vi "PyLoN_SRS4.vi"() -> ()   [LabVIEW 2014]
uses:
  <vilib>/Utility/file.llb/Write To Spreadsheet File (I64).vi
  <vilib>/Utility/file.llb/Write To Spreadsheet File (DBL).vi
panel:
  in  "CHEK ID":bool
  out "Max Value":dbl
  out "Min Value":dbl
  in  "Param ID":u32
  out "default value":dbl
  out "current value":dbl
  out "num of elements":dbl
  in  "?":bool
  in  "?":T1(tab)
  in  "Shutter State":u16(ring)=2 items=["Always Close", "Open Each Exposure", "Open Until Finish", "Open waiting for triger"]
  in  "Trigger Edge":u16(ring) items=["Positive", "Negative"]
  in  "Timing Mode":u16(ring) items=["Free Run", "Triger First", "Ext Sync", "Bulb Mode", "Variable Mode", "Flash Mode"]
  in  "ADC Speed":u16(ring)=2 items=["ADC Slowest", "ADC Fastest", "Default", "50 kHz", "100 kHz", "200 kHz", "500 kHz", "1 MHz"]
  in  "ADC Gain":u16(ring) items=["ADC Low", "ADC High"]
  in  "Temperature":dbl=-100.0 caption="SET Temperature" format="%.2f"
  in  "Skip Serial  Reg Clean":dbl=1.0 format="%.2f"
  in  "Vertical Timing":dbl=3.2
  out "Vertical Timing":dbl
  in  "Readout Port":i32=4 min=-1 step=1
  in  "?":T2={"X start"=0, "X end"=1023, "X Binning/Grouping"=1, "Y start"=0, "Y end"=1, "Y Binning/Grouping"=1}
  in  "Logic Out":u16(ring) items=["Not Scan", "Shutter", "Not Rady", "Logic 0", "Clearing", "Not Ft Image Shift", "Reserved", "Logic1", "Expos Prog", "Expos", "Image Shift", "Readout", "Acquiring", "Wait For Trig"]
  in  "Use Custom Chip":bool
  out "Readout Time":dbl caption="Readout time (ms)" format="%.2f"
  in  "Temp_bypass":bool
  in  "?":bool
  in  "Exposure Time (s)":dbl=0.004 min=0.0 step=0.001 format="%.3f"
  in  "?":bool
  in  "?":bool
  out "?":u16[](graph)
  in  "file path":path
  in  "File_name":string
  in  "# of spectrum per frame":i32
  in  "# of Frames":i32
  in  "FLIP SPECTRA":bool
  in  "?":bool
  in  "?":bool
  in  "?":bool
  out "?":dbl[](graph)
  in  "?":bool
  in  "Number of Images":u32=1 min=1 step=1
  out "?":dbl[](graph)
  in  "?":bool
  in  "# of Sets":i32
  out "Current Set":u32=24
  in  "#Ground per set":u32=3
  in  "Timepoints":dbl[](array[numeric])=[200.0, 100.0, 300.0, 400.0, 500.0]
  in  "File Path":path
  in  "File Name":string
  in  "Ground State\nSubstract?":bool
  in  "PyLonN Error In":errorcluster
  out "PyLoN Error Out":errorcluster
  out "PyLoN Ready":bool
  out "PyLoN \nTemperature":dbl
  # "REGION OF INTEREST"
  # "TRIGGER"
  # "ADC"
  # "SHUTTER"
  # "INPUT VARIABLES"
  # "TTL LOGIC"
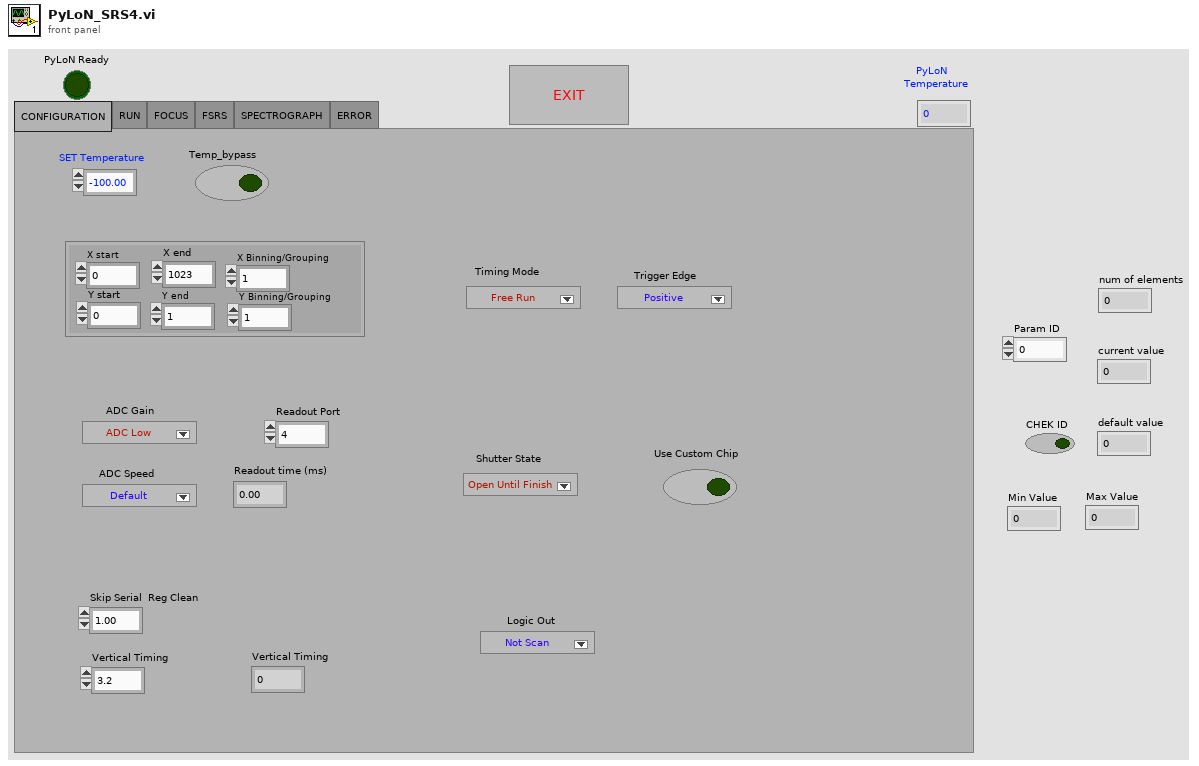
[diagram p1: front panel]
types:
  T1 = enum32{"CONFIGURATION", "RUN", "FOCUS", "FSRS", "SPECTROGRAPH", "ERROR"}
  T2 = cluster{"X start":u32, "X end":u32, "X Binning/Grouping":u32, "Y start":u32, "Y end":u32, "Y Binning/Grouping":u32}
  T3 = enum32{"Initializing", "RUN", "FSRS", "Monochromator", "Errors"}
  T4 = cluster{"Param ID":u32, "Avail Flag":u8, "Current Value":dbl, "Default Value":dbl, "Min Value":dbl, "Max Value":dbl, "Increment":dbl, "Data Type":u32, "Access Type":u32, "Bit Used Flag":u32, "Number of Enums":u32, "Description":string}
  T5 = cluster{"acquire focus mode":u32, "Exposure Time (s)":dbl, i32, "Software accumulation":u32}
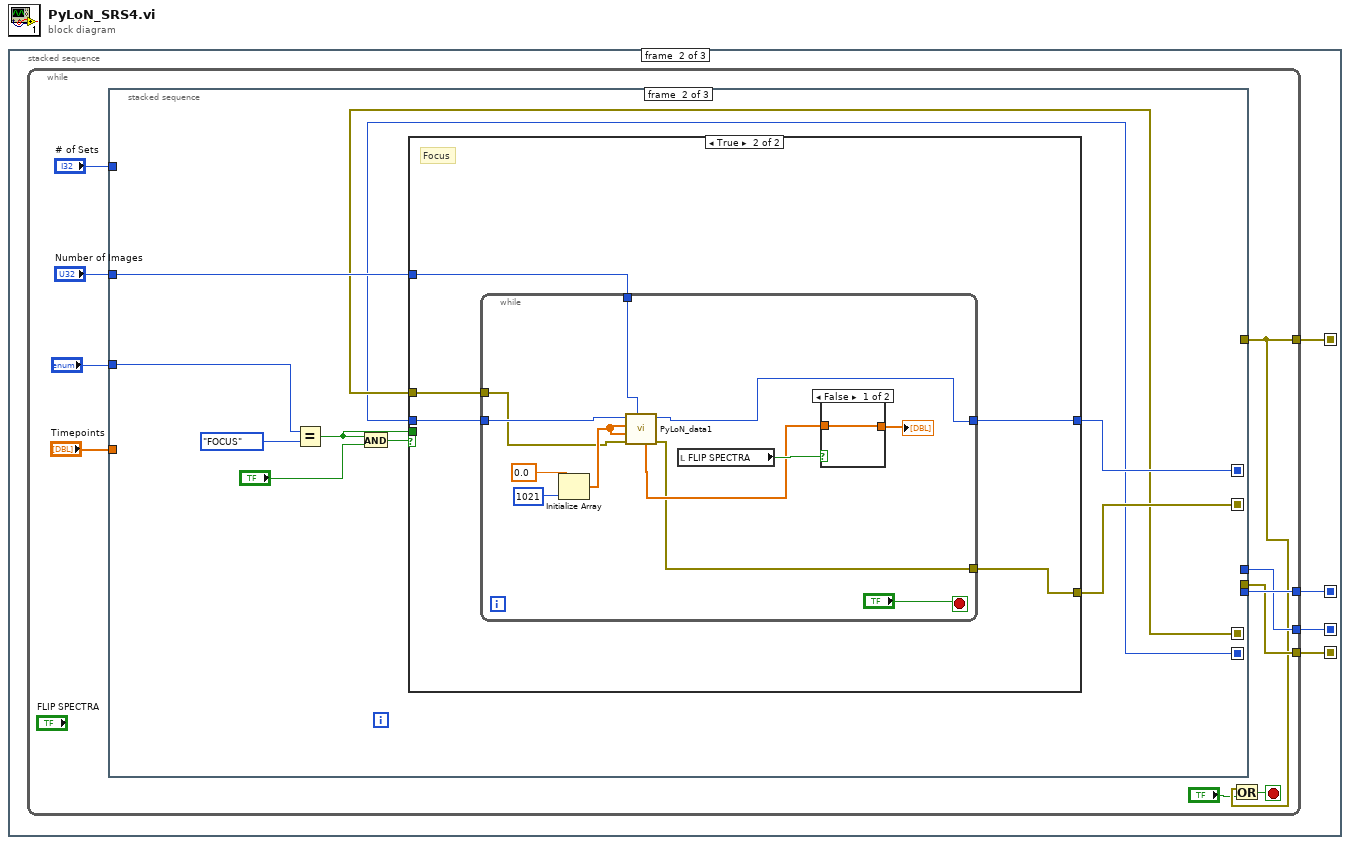
[diagram p0: block diagram]
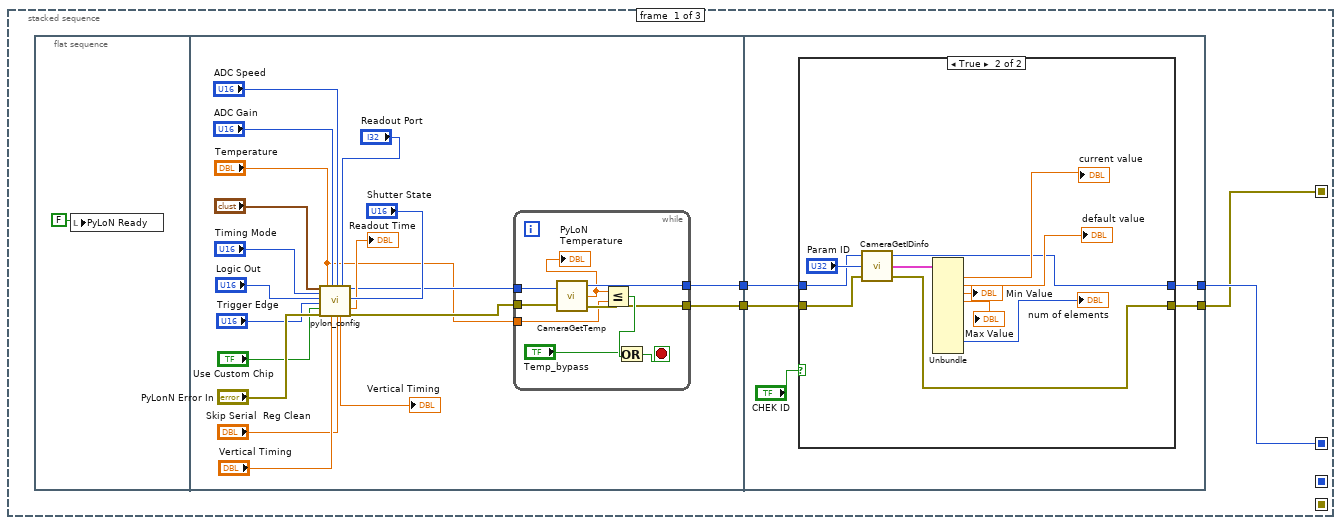
[diagram p2: hidden frame]
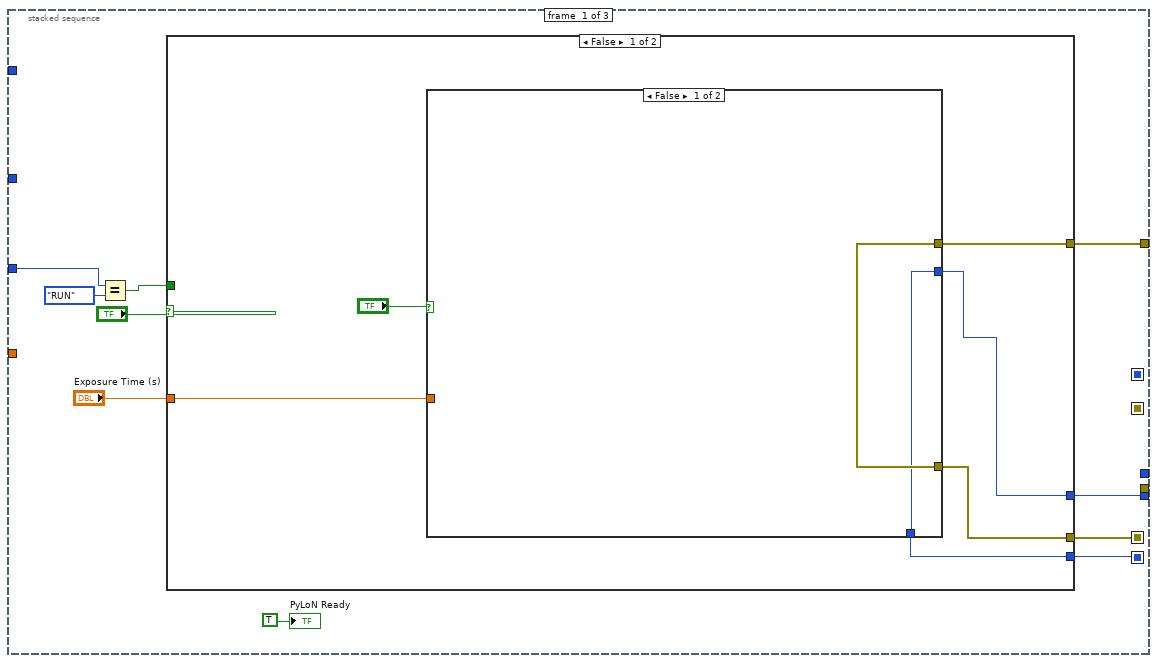
[diagram p4: hidden frame]
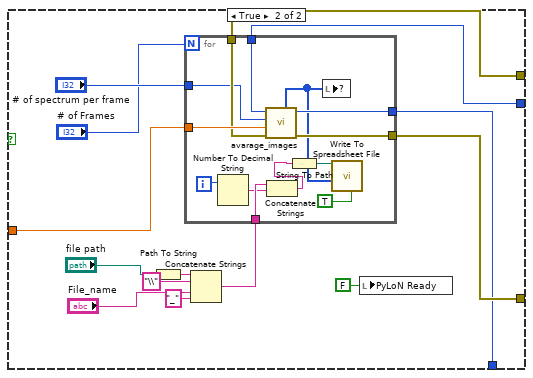
[diagram p5: hidden frame]
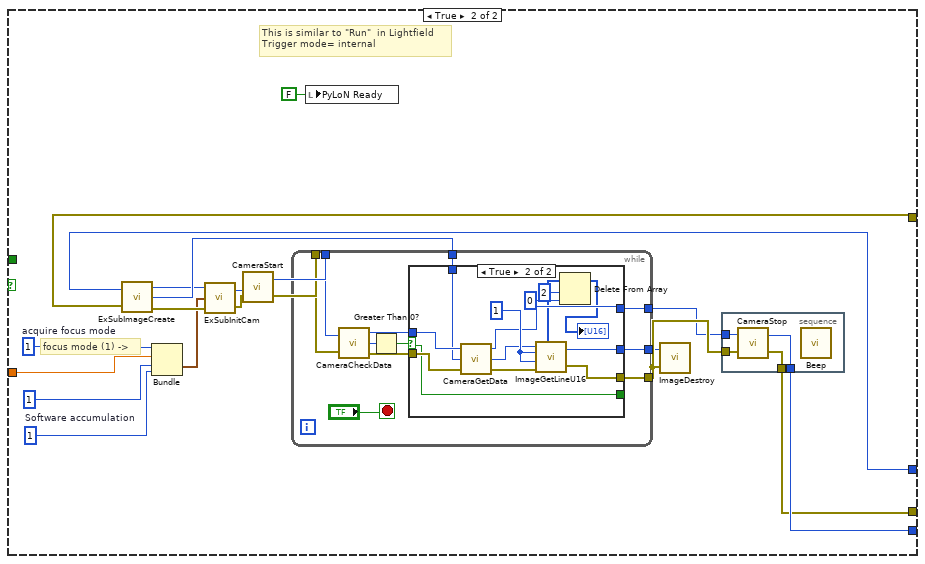
[diagram p6: hidden frame]
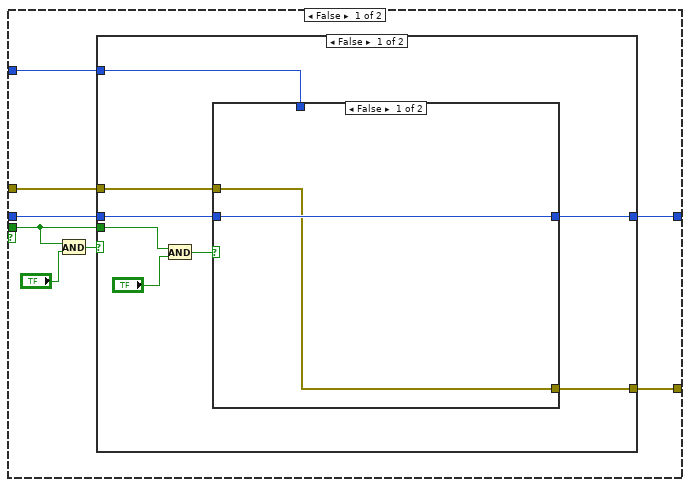
[diagram p8: hidden frame]
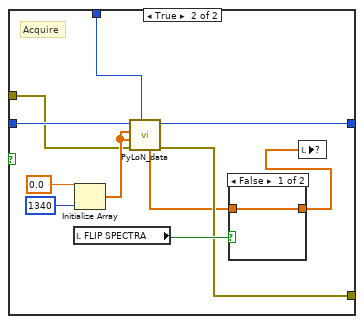
[diagram p9: hidden frame]
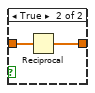
[diagram p10: hidden frame]
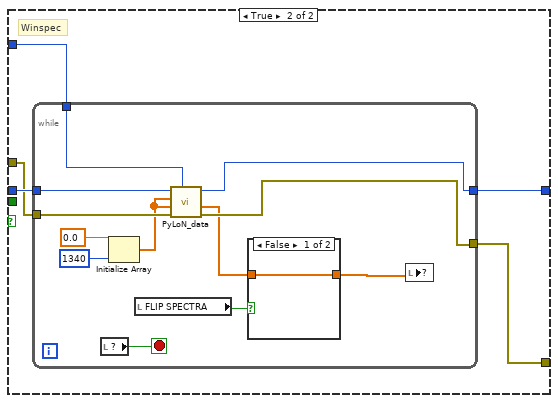
[diagram p11: hidden frame]
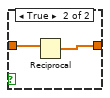
[diagram p12: hidden frame]
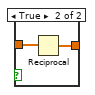
[diagram p13: hidden frame]
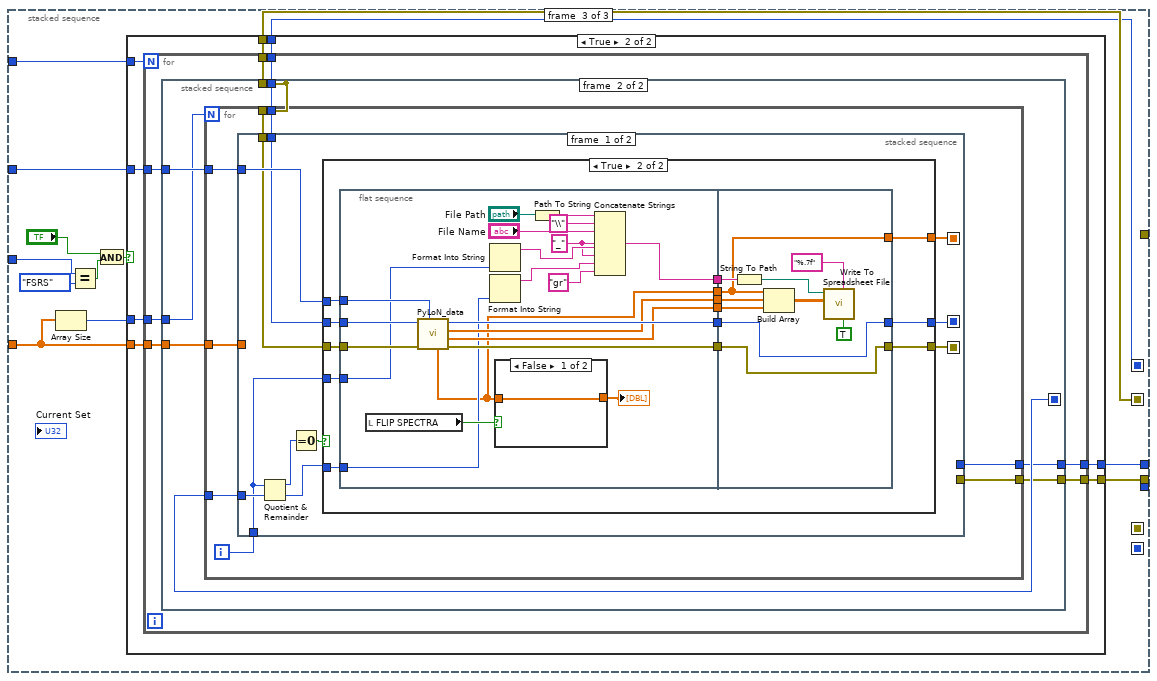
[diagram p14: hidden frame]
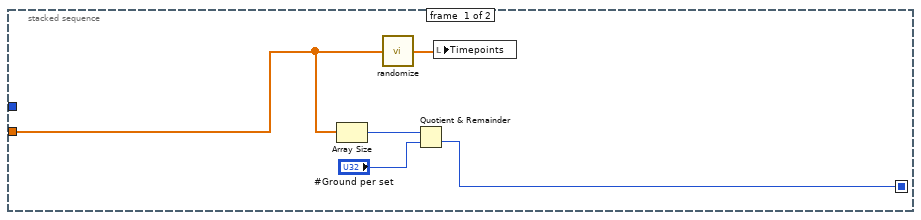
[diagram p16: hidden frame]
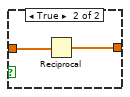
[diagram p18: hidden frame]
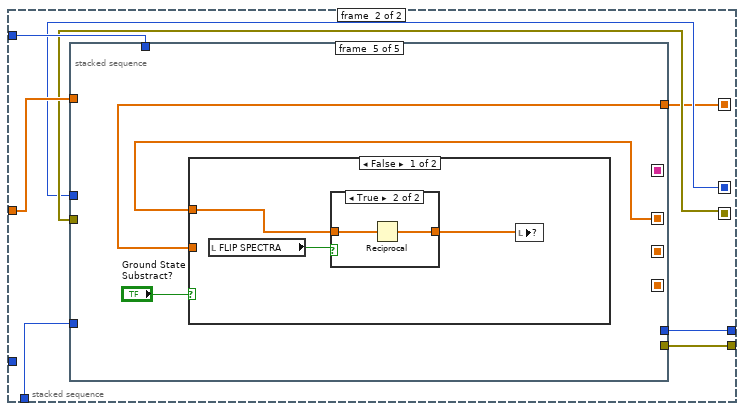
[diagram p19: hidden frame]
diagram:
  n1 = stacked-sequence {
    seq-local: [w3 _ _] -> [_ w52 _]
    seq-local: [w4 _ _] -> [_ w55 _]
    seq-local: [_ w54 _] -> [_ _ w416]
    seq-local: [_ w53 _] -> [_ _ w415]
    frame #0 {
      n2 = flat-sequence {
        tunnel: [w9] -> w2
        tunnel: [w7] -> w1
        tunnel: [w34] -> w3
        tunnel: [w37] -> w4
        tunnel: w2 -> [w38]
        tunnel: w1 -> [w36]
        frame #0 {
          n3 = local write "PyLoN Ready"(FALSE ("PyLoN Ready")) -> ()
        }
        frame #1 {
          n4 = call "pylon_config.vi"(0:"?", "Timing Mode"="Timing Mode", "Logic Out"="Logic Out", "Trigger Edge"="Trigger Edge", "Use Custom Chip"="Use Custom Chip", "PyLonN Error In"="PyLonN Error In", "Temperature"="Temperature", "ADC Gain"="ADC Gain", "Vertical Timing"="Vertical Timing", "ADC Speed"="ADC Speed", "Skip Serial  Reg Clean"="Skip Serial  Reg Clean", "Readout Port"="Readout Port", "Shutter State"="Shutter State") -> ("Vertical Timing"=→"Vertical Timing":dbl, "CameraHandle"=w10:u32, "Readout Time"=→"Readout Time":dbl, "error out"=w8:errorcluster)  [unwired: 3 in]
          n5 = while {
            tunnel: [w33] -> w9
            tunnel: w10 -> [w30]
            tunnel: w8 -> [w29]
            tunnel: [w28] -> w7
            tunnel: "Temperature" -> [w26]
            stop <- w32 stop-if-true
            n6 = call <userlib>:"CameraGetTemp.vi"("Camera Handle"=w30, "error in (no error)"=w29) -> ("Camera Handle"=w33:u32, "Temperature"=w27:dbl, "error out"=w28:errorcluster)
            "PyLoN \nTemperature" <- w27
            n7 = Less Or Equal?(x=w27, y=w26) -> (x <= y?=w31:bool)
            n8 = Or(x="Temp_bypass", y=w31) -> (x .or. y?=w32:bool)
          }
        }
        frame #2 {
          n9 = case shown="True" "CHEK ID" {
            tunnel: w38 -> [w40 w46]
            tunnel: [w40 w45] -> w37
            tunnel: w36 -> [w39 w44]
            tunnel: [w39 w43] -> w34
            frame False {
            }
            frame True {
              n10 = call <userlib>:"CameraGetIDinfo.vi"("error in"=w44, "Param ID"="Param ID", "Camera handle"=w46) -> ("error out"=w43:errorcluster, "Param ID Information"=w51:T4, "Camera handle"=w45:u32)
              n11 = Unbundle(w51) -> ("Current Value"=→"current value":dbl, "Default Value"=→"default value":dbl, "Min Value"=→"Min Value":dbl, "Max Value"=→"Max Value":dbl, "Number of Enums"=→"num of elements":u32)  [unwired: 7 out]
            }
          }
        }
      }
    }
    frame #1 {
      n12 = while {
        tunnel: w55 -> [w65]
        tunnel: w52 -> [w57]
        tunnel: [w61] -> w54
        tunnel: [w60] -> w53
        stop <- w58 stop-if-true
        n13 = stacked-sequence {
          seq-local: [_ w168 _] -> [_ _ w252]
          seq-local: [_ w167 _] -> [_ _ w254]
          seq-local: [w70 _ _] -> [_ w165 _]
          seq-local: [w71 _ _] -> [_ w166 _]
          tunnel: w65 -> [w68 _ _]
          tunnel: w57 -> [w75 _ _]
          tunnel: "?" -> [w72 w173 w258]
          tunnel: "Number of Images" -> [_ w171 w255]
          tunnel: "Timepoints" -> [_ _ w247]
          tunnel: [_ _ w251] -> w61
          tunnel: [_ _ w250] -> w60
          tunnel: "# of Sets" -> [_ _ w248]
          frame #0 {
            n14 = Equal?(x=w72, y=T3."RUN") -> (x = y?=w69:bool)
            n15 = case shown="False" "?" {
              tunnel: w75 -> [w81 w113]
              tunnel: [w78 w116] -> w70
              tunnel: [w80 w115] -> w71
              tunnel: w69 -> [_ _]
              tunnel: w68 -> [w79 w114]
              tunnel: "Exposure Time (s)" -> [w77 w111]
              frame False {
                n16 = case shown="False" "?" {
                  tunnel: w81 -> [w83 w95]
                  tunnel: [w83 w94] -> w80
                  tunnel: w79 -> [w82 w96]
                  tunnel: [w82 w93] -> w78
                  tunnel: w77 -> [_ w97]
                  frame False {
                  }
                  frame True {
                    n17 = Path To String(path="file path") -> (string=w89:string)
                    n18 = Concatenate Strings(w89, "\\" ("string"), "File_name", "_" ("string")) -> (w84:string)
                    n19 = for {
                      N: "# of Frames" -> [_]
                      tunnel: w97 -> [w110]
                      tunnel: w96 -> [w109]
                      tunnel: w95 -> [w108]
                      tunnel: [w107] -> w94
                      tunnel: [w106] -> w93
                      tunnel: "# of spectrum per frame" -> [w105]
                      tunnel: w84 -> [w101]
                      i -> [w98]
                      n20 = Number To Decimal String(number=w98) -> (decimal integer string=w100:string)  [unwired: 1 in]
                      n21 = call "avarage_images.vi"("error in (no error)"=w108, "Exposure Time (s)"=w110, "Number of Images"=w105, "Camera Handle"=w109) -> ("error out"=w107:errorcluster, "Camera Handle"=w106:u32, "Waveform Graph"=w104:i32[])  [unwired: 3 in, 2 out]
                      n22 = Concatenate Strings(w101, w100) -> (w99:string)
                      n23 = String To Path(string=w99) -> (path=w102:path)
                      n24 = local write item#9(w104) -> ()
                      n25 = call-poly <vilib>:"Write To Spreadsheet File.vi"("transpose? (no:F)"=TRUE, "1D data"=w104, "file path (dialog if empty)"=w102) -> ()  [unwired: 5 in, 1 out]
                    }
                    n26 = local write "PyLoN Ready"(FALSE ("PyLoN Ready")) -> ()
                  }
                }
              }
              frame True {
                w118 = u32 1  # acquire focus mode
                w119 = u32 1  # Software accumulation
                # "focus mode (1) ->"
                # "This is similar to \"Run\"  in Lightfield\nTrigger mode= internal"
                n27 = call "ExSubImageCreate.vi"("Camera Handle"=w114, "error in (no error)"=w113) -> ("Camera Handle"=w120:u32, "Data Handle"=w126:u32, "error out"=w121:errorcluster)
                n28 = Bundle("acquire focus mode"=w118, "Exposure Time (s)"=w111, 1, "Software accumulation"=w119) -> (w117:T5)  [unwired: 1 in]
                n29 = call "ExSubInitCam.vi"("error in (no error)"=w121, "Camera Information"=w117, "Camera Handle"=w120) -> ("error out"=w122:errorcluster, "Camera Handle"=w123:u32)
                n30 = call <userlib>:"CameraStart.vi"("error in"=w122, "Camera Handle"=w123) -> ("error out"=w124:errorcluster, "Camera Handle"=w125:u32)
                n31 = while {
                  tunnel: [w141] -> w127
                  tunnel: [w140] -> w129
                  tunnel: [w139] -> w128
                  tunnel: w124 -> [w138]
                  tunnel: w125 -> [w137]
                  tunnel: w126 -> [w136]
                  stop <- "?" stop-if-true
                  n32 = call <userlib>:"CameraCheckData.vi"("Camera Handle"=w137, "error in"=w138) -> ("Camera Handle"=w143:u32, "Number Of Frames Available"=w145:i32, "error out"=w142:errorcluster)
                  n33 = Greater Than 0?(x=w145) -> (x > 0?=w144:bool)
                  n34 = case shown="True" w144 {
                    selector: w144 -> [w148 w161]
                    tunnel: w143 -> [w146 w163]
                    tunnel: w142 -> [w149 w162]
                    tunnel: [w148 w161] -> _
                    tunnel: [w149 w160] -> w140
                    tunnel: w136 -> [w147 w154]
                    tunnel: [w147 w158] -> w141
                    tunnel: [w146 w157] -> w139
                    frame False {
                    }
                    frame True {
                      w159 = 1
                      n35 = call <userlib>:"CameraGetData.vi"("error in"=w162, "Data Handle"=w154, "Camera Handle"=w163) -> ("error out"=w156:errorcluster, "Data Handle"=w155:u32, "Camera Handle"=w157:u32)
                      n36 = call <userlib>:"ImageGetLineU16.vi"("Data Handle"=w155, "Y Position"=w159, "Z Position"=w159, "error in"=w156) -> ("Array u16"=w153:u16[], "Data Handle"=w158:u32, "error out"=w160:errorcluster)
                      n37 = Delete From Array(array=w153, length=2, index=0) -> (array with subset deleted=→"?":u16[])  [unwired: 1 out]
                    }
                  }
                }
                n38 = local write "PyLoN Ready"(FALSE ("PyLoN Ready")) -> ()
                n39 = call <userlib>:"ImageDestroy.vi"("error in"=w129, "Data handle"=w127) -> ()  [unwired: 1 out]
                n40 = stacked-sequence {
                  tunnel: w129 -> [w134]
                  tunnel: w128 -> [w133]
                  tunnel: [w132] -> w115
                  tunnel: [w131] -> w116
                  frame #0 {
                    n41 = call <userlib>:"CameraStop.vi"("error in"=w134, "Camera Handle"=w133) -> ("error out"=w132:errorcluster, "Camera Handle"=w131:u32)
                    n42 = call <vilib>:"Beep.vi"() -> ()  [unwired: 12 in]
                  }
                }
              }
            }
            "PyLoN Ready" <- TRUE
          }
          frame #1 {
            n43 = Equal?(x=w173, y=T1."FOCUS") -> (x = y?=w169:bool)
            n44 = And(x=w169, y="?") -> (x .and. y?=w172:bool)
            n45 = case shown="True" w172 {
              tunnel: w165 -> [w181 w230]
              tunnel: [w177 w229] -> w168
              tunnel: w166 -> [w179 w228]
              tunnel: w171 -> [w180 w227]
              tunnel: [w178 w226] -> w167
              tunnel: w169 -> [w174 _]
              frame False {
                n46 = And(x=w174, y="?") -> (x .and. y?=w176:bool)
                n47 = case shown="False" w176 {
                  tunnel: w181 -> [w184 w210]
                  tunnel: w180 -> [w185 w209]
                  tunnel: w179 -> [w186 w208]
                  tunnel: [w182 w207] -> w178
                  tunnel: [w183 w206] -> w177
                  tunnel: w174 -> [w187 _]
                  frame False {
                    n48 = And(x=w187, y="?") -> (x .and. y?=w189:bool)
                    n49 = case shown="False" w189 {
                      tunnel: w186 -> [w190 w195]
                      tunnel: w185 -> [_ w198]
                      tunnel: w184 -> [w191 w197]
                      tunnel: [w191 w193] -> w183
                      tunnel: [w190 w194] -> w182
                      frame False {
                      }
                      frame True {
                        # "Acquire"
                        n50 = local read "FLIP SPECTRA"() -> (w200:bool)
                        n51 = Initialize Array(0.0, u32 1340) -> (w196:dbl[])
                        n52 = call "PyLoN_data.vi"("Number of Images"=w198, "error in (no error)"=w195, "PumpOffBkgd"=w196, "PumpOnBkgd"=w196, "Camera Handle"=w197) -> ("error out"=w194:errorcluster, "Camera Handle 2"=w193:u32, "Raman_Gain"=w192:dbl[])  [unwired: 2 in, 2 out]
                        n53 = case shown="False" w200 {
                          tunnel: w192 -> [w203 w205]
                          tunnel: [w203 w204] -> w199
                          frame False {
                          }
                          frame True {
                            n54 = Reciprocal(x=w205) -> (1/x=w204:dbl[])
                          }
                        }
                        n55 = local write item#21(w199) -> ()
                      }
                    }
                  }
                  frame True {
                    # "Winspec"
                    n56 = while {
                      tunnel: w210 -> [w216]
                      tunnel: w209 -> [w217]
                      tunnel: [w211] -> w206
                      tunnel: w208 -> [w215]
                      tunnel: [w214] -> w207
                      stop <- w220 stop-if-true
                      n57 = local read item#27() -> (w220:bool)
                      n58 = Initialize Array(0.0, u32 1340) -> (w212:dbl[])
                      n59 = local read "FLIP SPECTRA"() -> (w219:bool)
                      n60 = call "PyLoN_data.vi"("Number of Images"=w217, "error in (no error)"=w215, "PumpOffBkgd"=w212, "PumpOnBkgd"=w212, "Camera Handle"=w216) -> ("error out"=w214:errorcluster, "Pump_Off"=w213:dbl[], "Camera Handle 2"=w211:u32)  [unwired: 2 in, 2 out]
                      n61 = case shown="False" w219 {
                        tunnel: w213 -> [w223 w224]
                        tunnel: [w223 w225] -> w218
                        frame False {
                        }
                        frame True {
                          n62 = Reciprocal(x=w224) -> (1/x=w225:dbl[])
                        }
                      }
                      n63 = local write item#21(w218) -> ()
                    }
                  }
                }
              }
              frame True {
                # "Focus"
                n64 = while {
                  tunnel: w228 -> [w234]
                  tunnel: w227 -> [w237]
                  tunnel: [w232] -> w226
                  tunnel: w230 -> [w236]
                  tunnel: [w231] -> w229
                  stop <- "?" stop-if-true
                  n65 = Initialize Array(0.0, u32 1021) -> (w235:dbl[])
                  n66 = call "PyLoN_data1.vi"("Number of Images"=w237, "error in (no error)"=w234, "PumpOffBkgd"=w235, "PumpOnBkgd"=w235, "Camera Handle"=w236) -> ("error out"=w232:errorcluster, "Camera Handle 2"=w231:u32, "Raman_Gain"=w233:dbl[])  [unwired: 2 in, 2 out]
                  n67 = local read "FLIP SPECTRA"() -> (w239:bool)
                  n68 = case shown="False" w239 {
                    tunnel: w233 -> [w243 w245]
                    tunnel: [w243 w244] -> w238
                    frame False {
                    }
                    frame True {
                      n69 = Reciprocal(x=w245) -> (1/x=w244:dbl[])
                    }
                  }
                  "?" <- w238
                }
              }
            }
          }
          frame #2 {
            n70 = Array Size(array=w247) -> (size(s)=w246:i32)
            n71 = Equal?(x=w258, y=T1."FSRS") -> (x = y?=w256:bool)
            n72 = And(x="?", y=w256) -> (x .and. y?=w257:bool)
            n73 = case shown="True" w257 {
              tunnel: w255 -> [_ w268]
              tunnel: w252 -> [w259 w267]
              tunnel: w254 -> [w260 w263]
              tunnel: w247 -> [_ w266]
              tunnel: [w259 w265] -> w251
              tunnel: [w260 w264] -> w250
              tunnel: w248 -> [_ w262]
              tunnel: w246 -> [_ w261]
              frame False {
              }
              frame True {
                n74 = for {
                  N: w262 -> [_]
                  tunnel: w268 -> [w275]
                  tunnel: w267 -> [w274]
                  tunnel: w266 -> [w273]
                  tunnel: [w272] -> w265
                  tunnel: [w271] -> w264
                  tunnel: w263 -> [w270]
                  tunnel: w261 -> [w269]
                  n75 = stacked-sequence {
                    seq-local: [w278 _] -> [_ w288]
                    tunnel: w275 -> [_ w287]
                    tunnel: w274 -> [_ w286]
                    tunnel: [_ w282] -> _
                    tunnel: w273 -> [w276 w285]
                    tunnel: [_ w284] -> w271
                    tunnel: [_ w283] -> w272
                    tunnel: w270 -> [_ w282]
                    tunnel: w269 -> [_ w281]
                    frame #0 {
                      n76 = Array Size(array=w276) -> (size(s)=w280:i32)
                      n77 = call "randomize.vi"("Input array"=w276) -> ("Output array"=w277:dbl[])
                      n78 = Quotient & Remainder(x=w280, y="#Ground per set") -> (floor(x/y)=w278:u32)  [unwired: 1 out]
                      n79 = local write "Timepoints"(w277) -> ()
                    }
                    frame #1 {
                      n80 = for {
                        N: w281 -> [_]
                        tunnel: w288 -> [w295]
                        tunnel: w287 -> [w294]
                        tunnel: w286 -> [w293]
                        tunnel: w285 -> [w292]
                        tunnel: [w291] -> w284
                        tunnel: [w290] -> w283
                        tunnel: w282 -> [w289]
                        i -> [w296]
                        n81 = stacked-sequence {
                          seq-local: [w298 _] -> [_ w361]
                          seq-local: [w299 _] -> [_ w362]
                          seq-local: [w297 _] -> [_ w360]
                          tunnel: w296 -> [w300 w363]
                          tunnel: w295 -> [w305 _]
                          tunnel: w294 -> [w303 w365]
                          tunnel: w293 -> [w302 _]
                          tunnel: w289 -> [w301 _]
                          tunnel: w292 -> [_ w364]
                          tunnel: [_ w359] -> w291
                          tunnel: [_ w358] -> w290
                          frame #0 {
                            n82 = Quotient & Remainder(x=w300, y=w305) -> (x-y*floor(x/y)=w306:u32, floor(x/y)=w304:u32)
                            n83 = Equal To 0?(x=w306) -> (x = 0?=w307:bool)
                            n84 = case shown="True" w307 {
                              tunnel: w304 -> [_ w319]
                              tunnel: w303 -> [_ w323]
                              tunnel: w302 -> [w309 w322]
                              tunnel: w301 -> [w308 w321]
                              tunnel: [w309 w312] -> w298
                              tunnel: [w308 w311] -> w299
                              tunnel: w300 -> [_ w320]
                              tunnel: [_ w310] -> w297
                              frame False {
                              }
                              frame True {
                                n85 = flat-sequence {
                                tunnel: w323 -> [w344]
                                tunnel: w322 -> [w343]
                                tunnel: w321 -> [w342]
                                tunnel: w320 -> [w330]
                                tunnel: w319 -> [w328]
                                tunnel: [w341] -> w318
                                tunnel: [w340] -> w317
                                tunnel: [w337] -> w316
                                tunnel: [w336] -> w315
                                tunnel: [w325] -> w314
                                tunnel: [w324] -> w313
                                tunnel: w318 -> [w350]
                                tunnel: w317 -> [w349]
                                tunnel: w316 -> [w353]
                                tunnel: w315 -> [w352]
                                tunnel: w314 -> [w354]
                                tunnel: w313 -> [w348]
                                tunnel: [w350] -> w312
                                tunnel: [w349] -> w311
                                tunnel: [w348] -> w310
                                frame #0 {
                                w329 = "_" ("string")
                                n86 = local read "FLIP SPECTRA"() -> (w339:bool)
                                n87 = call "PyLoN_data.vi"("Number of Images"=w344, "error in (no error)"=w342, "Camera Handle"=w343) -> ("error out"=w340:errorcluster, "Pump_Off"=w336:dbl[], "Pump_On"=w337:dbl[], "Camera Handle 2"=w341:u32, "Raman_Gain"=w324:dbl[])  [unwired: 4 in]
                                n88 = Format Into String(w330) -> (resulting string=w331:string)  [unwired: 3 in, 1 out]
                                n89 = Format Into String(w328) -> (resulting string=w327:string)  [unwired: 3 in, 1 out]
                                n90 = case shown="False" w339 {
                                tunnel: w324 -> [w345 w347]
                                tunnel: [w345 w346] -> w338
                                frame False {
                                }
                                frame True {
                                n91 = Reciprocal(x=w347) -> (1/x=w346:dbl[])
                                }
                                }
                                "?" <- w338
                                n92 = Path To String(path="File Path") -> (string=w335:string)
                                n93 = Concatenate Strings(w335, "\\" ("string"), "File Name", w329, w331, w329, w327, "gr" ("string")) -> (w325:string)
                                }
                                frame #1 {
                                n94 = String To Path(string=w354) -> (path=w355:path)
                                n95 = Build Array(w348, w353, w352) -> (w351:dbl[][])
                                n96 = call-poly <vilib>:"Write To Spreadsheet File.vi"("transpose? (no:F)"=TRUE, "format (%.3f)"="%.7f", "2D data"=w351, "file path (dialog if empty)"=w355) -> ()  [unwired: 4 in, 1 out]
                                }
                                }
                              }
                            }
                          }
                          frame #1 {
                            n97 = stacked-sequence {
                              seq-local: [_ w368 _ _ _] -> [_ _ _ w389 _]
                              seq-local: [_ w371 _ _ _] -> [_ _ _ w388 w395]
                              seq-local: [_ w370 _ _ _] -> [_ _ _ w387 _]
                              seq-local: [_ w369 _ _ _] -> [_ _ _ w386 _]
                              tunnel: w362 -> [_ w381 _ _ _]
                              tunnel: w361 -> [_ w380 _ _ _]
                              tunnel: w365 -> [_ w379 _ _ _]
                              tunnel: w364 -> [_ w376 _ _ _]
                              tunnel: w363 -> [_ w372 _ _ _]
                              tunnel: w360 -> [_ _ _ _ w396]
                              tunnel: [_ w367 _ _ _] -> w359
                              tunnel: [_ w366 _ _ _] -> w358
                              frame #0 {
                              }
                              frame #1 {
                                n98 = Index Array(array=w376, index=w372) -> (element=w375:dbl)
                                n99 = call "tppathcr.vi"("input"=w375) -> ("out"=w374:string)
                                n100 = local read "File Path"() -> (w378:path)
                                n101 = local read "File Name"() -> (w377:string)
                                n102 = call "PyLoN_data.vi"("Number of Images"=w379, "error in (no error)"=w381, "Camera Handle"=w380) -> ("error out"=w367:errorcluster, "Pump_Off"=w369:dbl[], "Pump_On"=w370:dbl[], "Camera Handle 2"=w366:u32, "Raman_Gain"=w371:dbl[])  [unwired: 4 in]
                                n103 = Format Into String(w372) -> (resulting string=w382:string)  [unwired: 3 in, 1 out]
                                n104 = Path To String(path=w378) -> (string=w385:string)
                                n105 = Concatenate Strings(w385, "\\" ("string"), w377, "_" ("string"), w374, "exe" ("string"), w382) -> (w368:string)
                              }
                              frame #2 {
                              }
                              frame #3 {
                                n106 = String To Path(string=w389) -> (path=w391:path)
                                n107 = Build Array(w388, w387, w386) -> (w390:dbl[][])
                                n108 = call-poly <vilib>:"Write To Spreadsheet File.vi"("transpose? (no:F)"=TRUE, "format (%.3f)"="%.7f", "2D data"=w390, "file path (dialog if empty)"=w391) -> ()  [unwired: 4 in, 1 out]
                              }
                              frame #4 {
                                n109 = case shown="False" "Ground State\nSubstract?" {
                                tunnel: w396 -> [_ w405]
                                tunnel: w395 -> [w399 w404]
                                frame False {
                                n110 = local read "FLIP SPECTRA"() -> (w398:bool)
                                n111 = case shown="True" w398 {
                                tunnel: [w400 w402] -> w397
                                tunnel: w399 -> [w400 w401]
                                frame False {
                                }
                                frame True {
                                n112 = Reciprocal(x=w401) -> (1/x=w402:dbl[])
                                }
                                }
                                n113 = local write item#33(w397) -> ()
                                }
                                frame True {
                                n114 = local read "FLIP SPECTRA"() -> (w406:bool)
                                n115 = case shown="False" w406 {
                                tunnel: [w409 w414] -> w408
                                tunnel: w405 -> [w410 w411]
                                tunnel: [w410 w413] -> w407
                                tunnel: w404 -> [w409 w412]
                                frame False {
                                }
                                frame True {
                                n116 = Reciprocal(x=w412) -> (1/x=w414:dbl[])
                                n117 = Reciprocal(x=w411) -> (1/x=w413:dbl[])
                                }
                                }
                                n118 = Subtract(x=w408, y=w407) -> (x-y=w403:dbl[])
                                n119 = local write item#33(w403) -> ()
                                }
                                }
                              }
                            }
                          }
                        }
                      }
                    }
                  }
                }
              }
            }
          }
        }
        n120 = Or(x=w57, y="?") -> (x .or. y?=w58:bool)
      }
    }
    frame #2 {
      n121 = local write "PyLoN Ready"(FALSE ("PyLoN Ready")) -> ()
      n122 = call "ExSubCloseCamUnInit.vi"("error in (no error)"=w415, "Camera Handle"=w416) -> ("error out"=→"PyLoN Error Out":errorcluster)
    }
  }
